vi "Build [5,5] Reference Array.vi"(8 "error in":errorcluster {"code" format="%.0x"}, 11 "controls references":refnum<vi>[](array[refnum])) -> (0 "error out":errorcluster {"code" format="%.0x"}, 2 "2-D controls references array":refnum<vi>[][](array[refnum]), 3 "controls references out":refnum<vi>[](array[refnum]))   [LabVIEW 2018, in "NISAST VI Scripting.lvlib" / "VI.lvlib" / "Front Panel.lvlib"]
uses:
  Front Panel.lvlib
panel:
  in  "indicators initalize":refnum<vi>[](array[refnum])
  in  "controls initalize":refnum<vi>[](array[refnum])
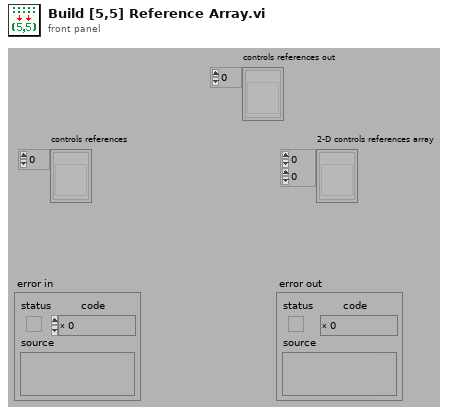
[diagram p1: front panel]
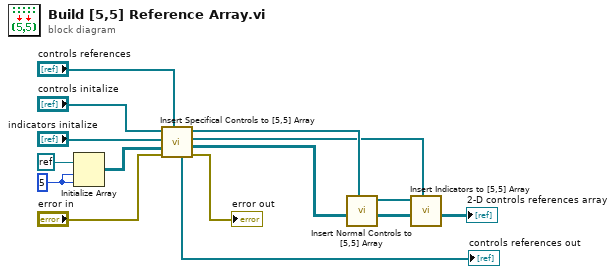
[diagram p0: block diagram]
diagram:
  w15 = 5 ("Dimension Size")
  n1 = Initialize Array(refnum<k0> refnum, w15, w15) -> (w10:refnum<k0>[][])
  n2 = call "Insert Specifical Controls to [5,5] Array.vi"("controls references"="controls references", "error in"="error in", "2-D controls references"=w10, "indicators"="indicators initalize", "controls"="controls initalize") -> ("error out"=→"error out":errorcluster, "2-D controls references out"=w4:refnum<vi>[][], "indicators out"=w7:refnum<vi>[], "controls out"=w8:refnum<vi>[], "controls references out"=→"controls references out":refnum<vi>[])  [unwired: 2 out]
  n3 = call "Insert Normal Controls to [5,5] Array.vi"("controls"=w8, "2-D controls references"=w4) -> ("2-D controls references out"=w3:refnum<vi>[][], "controls out"=w1:refnum<vi>[])  [unwired: 8 out]
  n4 = call "Insert Indicators to [5,5] Array.vi"("indicators"=w7, "2-D controls references"=w3, "controls"=w1) -> ("2-D controls references out"=→"2-D controls references array":refnum<vi>[][])  [unwired: 8 out]
